vi "Update State.vi"(8 "error in (no error)":errorcluster, 11 "Car Wash Controller Actor in":refnum<class "Car Wash Controller Actor.lvclass">) -> (0 "error out":errorcluster, 3 "Car Wash Controller Actor out":refnum<class "Car Wash Controller Actor.lvclass">)   [LabVIEW 2019]
uses:
  <vilib>/ActorFramework/Actor/Actor.lvclass
  Simulated Wash Display Console Actor/Simulated Wash Display Console Actor/Simulated Wash Display Console Actor.lvclass
  Sim Entry Console Actor/Sim Entry Console Actor/Wash steps selection -Buttons.ctl
  Sim Entry Console Actor/Sim Entry Console Actor/Simulated Entry Console Actor.lvclass
  Vehicle Position Simulation/Vehicle Position Simulation/Vehicle Position Simulation.lvclass
  Car Wash Controller Actor Messages/Set State Msg/Set State Msg.lvclass
  State -Enum.ctl
  Car Wash Controller Actor.lvclass
  C:/Program Files (x86)/National Instruments/LabVIEW 2019/vi.lib/ActorFramework/Actor/Actor.lvclass
  C:/Workspace/CLA/Carwasher AF/Abstract Entry Console Actor/Abstract Entry Console Actor/Entry Console Actor.lvclass
  C:/Workspace/CLA/Carwasher AF/Abstract Washer Display Console Actor/Abstract Washer Display Console Actor/Washer Display Console Actor.lvclass
  C:/Workspace/CLA/Carwasher AF/Abstract Vehicle Position Interface/Abstract Vehicle Position Interface/Vehicle Position Interface.lvclass
  Simulated Configuration Database Actor/Simulated Configuration Database Actor/Simulated Configuration Database Actor.lvclass
  C:/Workspace/CLA/Carwasher AF/Configuration Database Actor/Configuration Database Actor/Configuration Database Actor.lvclass
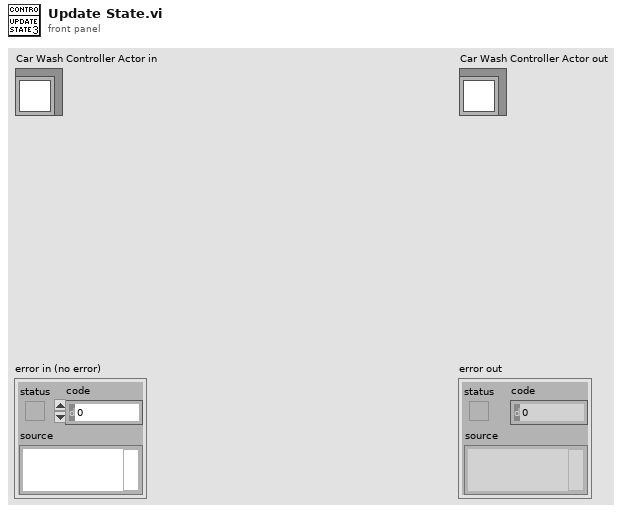
[diagram p1: front panel]
types:
  T1 = typedef "Car Wash Controller Actor.lvlib/Car Wash Controller Actor.lvclass/State -Enum.ctl" = enum16{"Initial", "Wait for Start", "Start", "Wait for Vehicle Position", "Wash Step Execution", "Wash Step/Cycle Completion", "Wash Exit", "Wash Abort/Terminate"}
  T2 = typedef "Simulated Entry Console Actor.lvlib/Simulated Entry Console Actor.lvclass/Wash steps selection -Buttons.ctl" = cluster{"Under Body Wash":bool, "Bug Remover":bool, "Pre-Soak":bool, "High Pressure Wash (default)":bool, "Low Pressure Wax":bool, "Spot Free Rinse":bool, "Tire Shine Foam":bool, "Air Dry":bool}
  T3 = enum8{"Enabled", "Disabled", "Disabled and Grayed Out"}
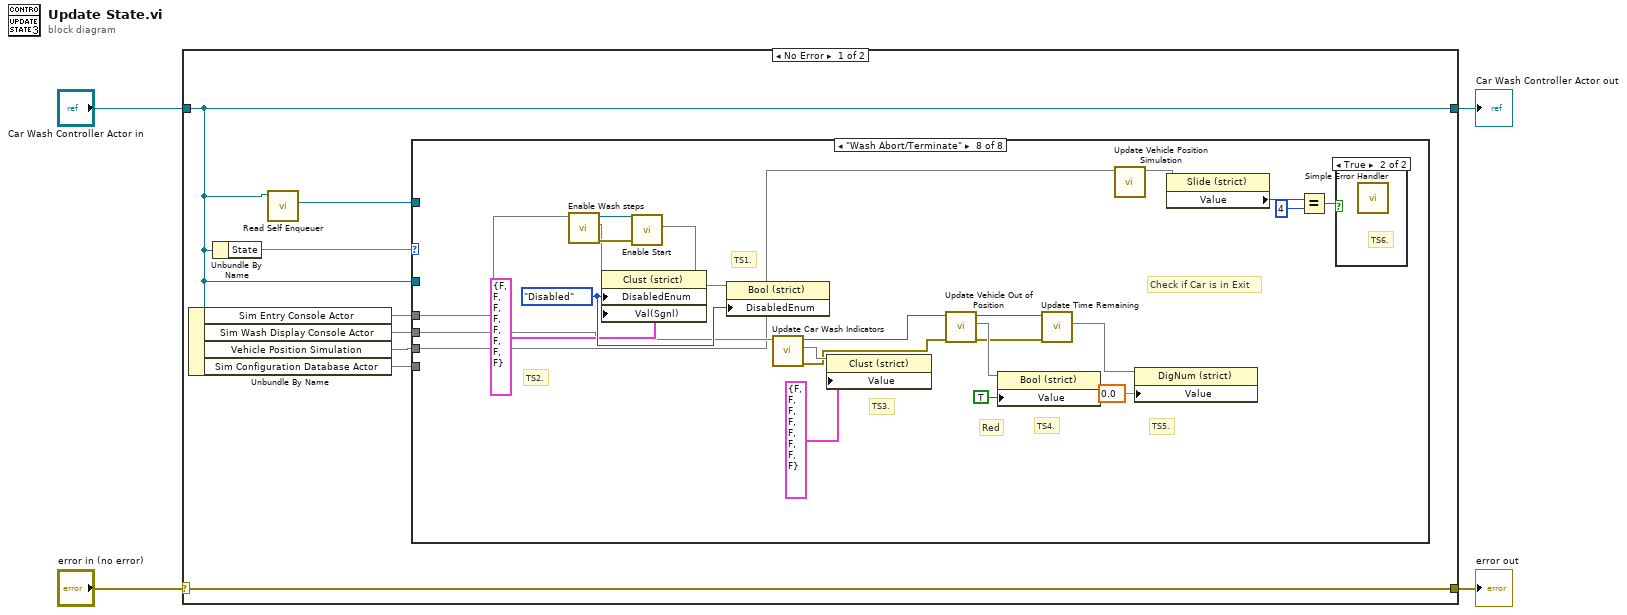
[diagram p0: block diagram]
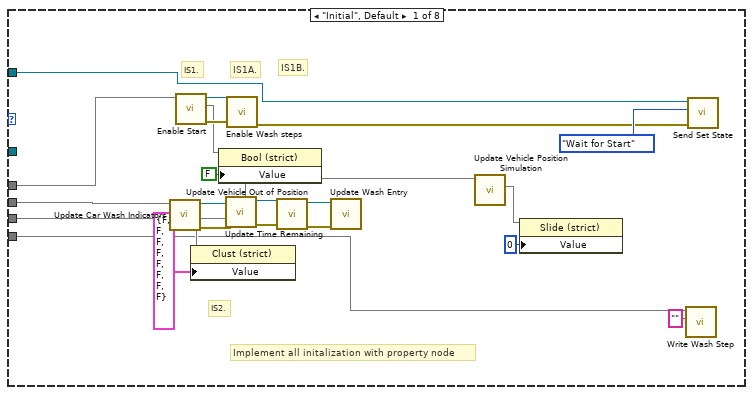
[diagram p2: hidden frame]
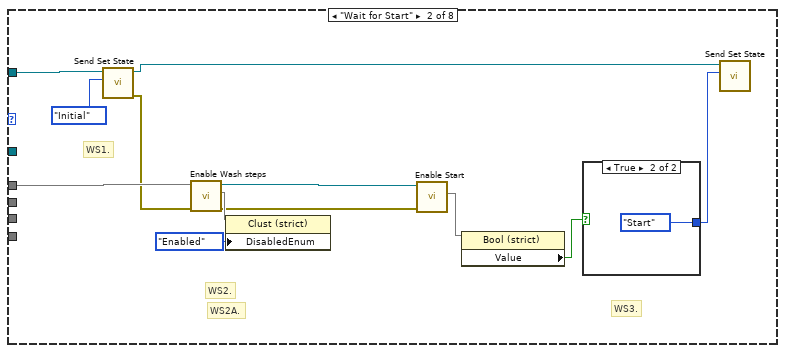
[diagram p3: hidden frame]
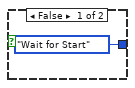
[diagram p4: hidden frame]
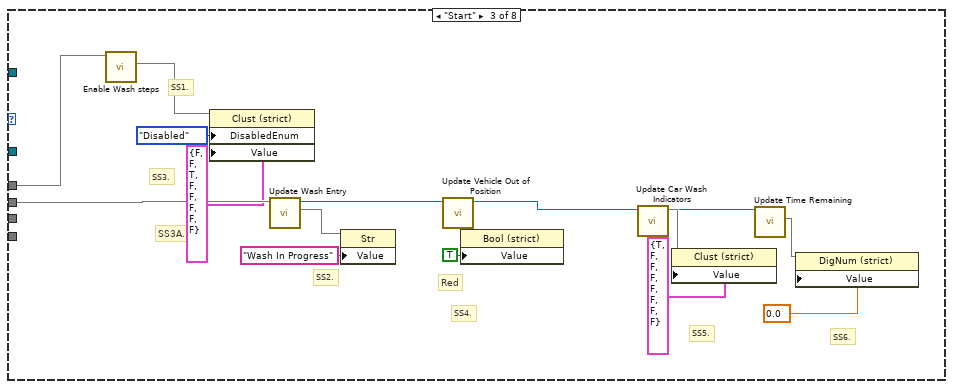
[diagram p5: hidden frame]
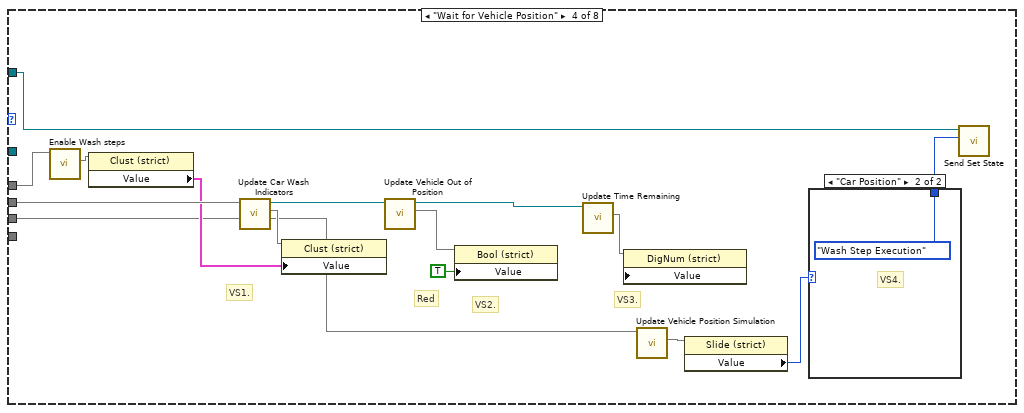
[diagram p6: hidden frame]
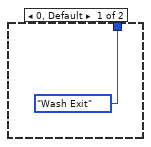
[diagram p7: hidden frame]
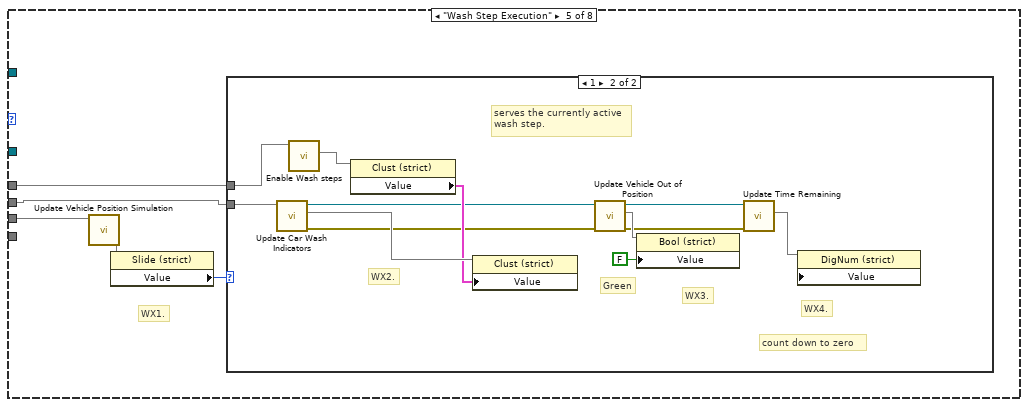
[diagram p8: hidden frame]
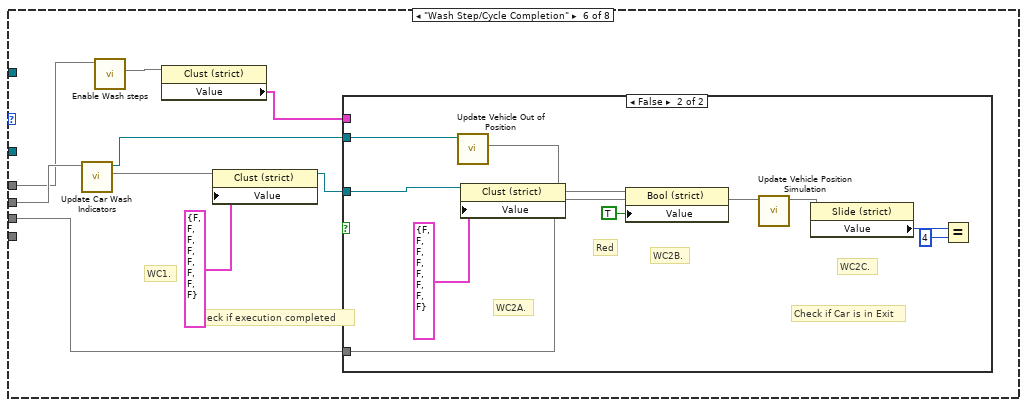
[diagram p10: hidden frame]
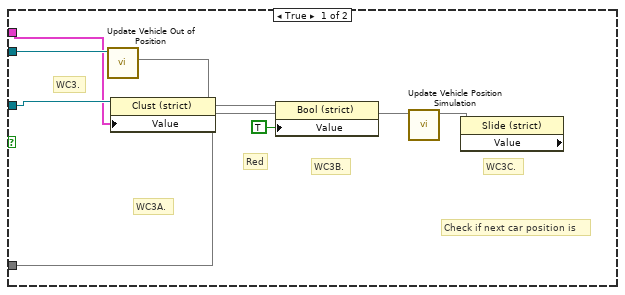
[diagram p11: hidden frame]
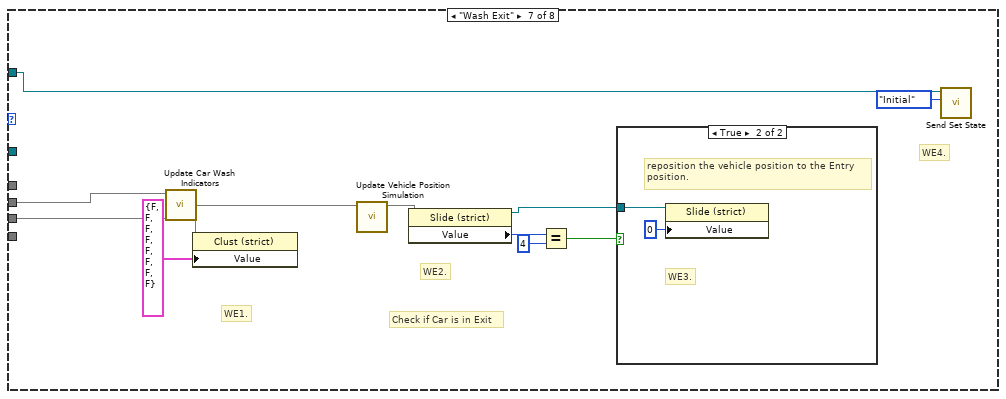
[diagram p12: hidden frame]
diagram:
  n1 = case shown="No Error" "error in (no error)" {
    selector: "error in (no error)" -> [w12 w161]
    tunnel: [w12 w161] -> w3
    tunnel: [w5 w160] -> w1
    tunnel: "Car Wash Controller Actor in" -> [w5 w160]
    frame No Error {
      n2 = Unbundle By Name(w5) -> ("Sim Entry Console Actor"=w9, "Sim Wash Display Console Actor"=w8, "Vehicle Position Simulation"=w7, "Sim Configuration Database Actor"=w6)
      n3 = Unbundle By Name(w5) -> ("State"=w11)
      n4 = call <vilib>:"Read Self Enqueuer.vi"("Actor"=w5) -> ("Self Enqueuer"=w10:refnum<class "Message Enqueuer.lvclass">)  [unwired: 10 in]
      n5 = case shown="\"Wash Abort/Terminate\"" w11 {
        tunnel: w10 -> [w15 w46 _ w66 _ _ w125 _]
        tunnel: w9 -> [w23 w44 w64 w77 w82 w101 _ w157]
        tunnel: w8 -> [w34 _ w61 w79 w83 w106 w134 w152]
        tunnel: w7 -> [w20 _ _ w69 w86 w102 w128 w138]
        tunnel: w6 -> [w17 _ _ _ _ _ _ _]
        tunnel: w5 -> [_ _ _ _ _ _ _ _]
        frame "Initial", Default {
          # "IS2."
          # "Implement all initalization with property node"
          # "IS1B."
          # "IS1A."
          # "IS1."
          n6 = call "Update Car Wash Indicators.vi"("Simulated Wash Display Console Actor in"=w34) -> ("error out"=w30:errorcluster, 2:w27, "Simulated Wash Display Console Actor out"=w33:refnum<class "Simulated Wash Display Console Actor.lvclass">)  [unwired: 8 in]
          n7 = call "Enable Start.vi"("Simulated Entry Console Actor in"=w23) -> ("error out"=w24:errorcluster, 2:w22, "Simulated Entry Console Actor out"=w25:refnum<class "Simulated Entry Console Actor.lvclass">)  [unwired: 8 in]
          n8 = property class="Clust (strict)"(reference=w27, "Value"=T2 {"Under Body Wash"=FALSE, "Bug Remover"=FALSE, "Pre-Soak"=FALSE, "High Pressure Wash (default)"=FALSE, "Low Pressure Wax"=FALSE, "Spot Free Rinse"=FALSE, "Tire Shine Foam"=FALSE, "Air Dry"=FALSE}) -> ()  [unwired: 1 in, 2 out]
          n9 = property class="Bool (strict)"(reference=w22, "Value"=FALSE) -> ()  [unwired: 1 in, 2 out]
          n10 = call "Update Time Remaining.vi"("error in (no error)"=w30, "Simulated Wash Display Console Actor in"=w33) -> ("error out"=w29:errorcluster, "Simulated Wash Display Console Actor out"=w32:refnum<class "Simulated Wash Display Console Actor.lvclass">)  [unwired: 8 in]
          n11 = call "Enable Wash steps.vi"("error in (no error)"=w24, "Simulated Entry Console Actor in"=w25) -> ("error out"=w13:errorcluster)  [unwired: 8 in, 1 out]
          n12 = call "Update Vehicle Out of Position.vi"("error in (no error)"=w29, "Simulated Wash Display Console Actor in"=w32) -> ("error out"=w28:errorcluster, "Simulated Wash Display Console Actor out"=w31:refnum<class "Simulated Wash Display Console Actor.lvclass">)  [unwired: 8 in]
          n13 = call "Update Wash Entry.vi"("error in (no error)"=w28, "Simulated Wash Display Console Actor in"=w31) -> ()  [unwired: 8 in, 2 out]
          n14 = call "Update Vehicle Position Simulation.vi"("Vehicle Position Simulation in"=w20) -> (2:w19)  [unwired: 8 in, 2 out]
          n15 = property class="Slide (strict)"(reference=w19, "Value"=u32 0) -> ()  [unwired: 1 in, 2 out]
          n16 = call-dynamic "Write Wash Step.vi"("Wash Step"="", "Simulated Configuration Database Actor in"=w17) -> ()  [unwired: 8 in, 2 out]
          n17 = call "Send Set State.vi"("error in (no error)"=w13, "States"=State_-Enum."Wait for Start", "Message Enqueuer"=w15) -> ()  [unwired: 7 in, 2 out]
        }
        frame "Wait for Start" {
          # "WS3."
          # "WS2A."
          # "WS2."
          # "WS1."
          n18 = call "Send Set State.vi"("States"=State_-Enum."Initial", "Message Enqueuer"=w46) -> ("error out"=w38:errorcluster, "Message Enqueuer out"=w36:refnum<class "Message Enqueuer.lvclass">)  [unwired: 8 in]
          n19 = call "Enable Wash steps.vi"("error in (no error)"=w38, "Simulated Entry Console Actor in"=w44) -> ("error out"=w37:errorcluster, 2:w43, "Simulated Entry Console Actor out"=w41:refnum<class "Simulated Entry Console Actor.lvclass">)  [unwired: 7 in]
          n20 = property class="Clust (strict)"(reference=w43, "DisabledEnum"=T3."Enabled" ("Disabled")) -> ()  [unwired: 1 in, 2 out]
          n21 = call "Enable Start.vi"("error in (no error)"=w37, "Simulated Entry Console Actor in"=w41) -> (2:w40)  [unwired: 7 in, 2 out]
          n22 = property class="Bool (strict)"(reference=w40) -> ("Value"=w39:bool)  [unwired: 1 in, 2 out]
          n23 = case shown="True" w39 {
            tunnel: [State_-Enum."Wait for Start" ("States") State_-Enum."Start" ("States")] -> w35
            frame False {
            }
            frame True {
            }
          }
          n24 = call "Send Set State.vi"("States"=w35, "Message Enqueuer"=w36) -> ()  [unwired: 8 in, 2 out]
        }
        frame "Start" {
          # "SS6."
          # "SS5."
          # "SS4."
          # "Red"
          # "SS3A."
          # "SS3."
          # "SS2."
          # "SS1."
          n25 = call "Enable Wash steps.vi"("Simulated Entry Console Actor in"=w64) -> (2:w63)  [unwired: 8 in, 2 out]
          n26 = property class="Clust (strict)"(reference=w63, "DisabledEnum"=T3."Disabled" ("Disabled"), "Value"=T2 {"Under Body Wash"=FALSE, "Bug Remover"=FALSE, "Pre-Soak"=TRUE, "High Pressure Wash (default)"=FALSE, "Low Pressure Wax"=FALSE, "Spot Free Rinse"=FALSE, "Tire Shine Foam"=FALSE, "Air Dry"=FALSE}) -> ()  [unwired: 1 in, 2 out]
          n27 = call "Update Wash Entry.vi"("Simulated Wash Display Console Actor in"=w61) -> (2:w60, "Simulated Wash Display Console Actor out"=w57:refnum<class "Simulated Wash Display Console Actor.lvclass">)  [unwired: 8 in, 1 out]
          n28 = property class="Str"(reference=w60, "Value"="Wash In Progress") -> ()  [unwired: 1 in, 2 out]
          n29 = call "Update Vehicle Out of Position.vi"("Simulated Wash Display Console Actor in"=w57) -> (2:w56, "Simulated Wash Display Console Actor out"=w54:refnum<class "Simulated Wash Display Console Actor.lvclass">)  [unwired: 8 in, 1 out]
          n30 = property class="Bool (strict)"(reference=w56, "Value"=TRUE) -> ()  [unwired: 1 in, 2 out]
          n31 = call "Update Car Wash Indicators.vi"("Simulated Wash Display Console Actor in"=w54) -> (2:w53, "Simulated Wash Display Console Actor out"=w51:refnum<class "Simulated Wash Display Console Actor.lvclass">)  [unwired: 8 in, 1 out]
          n32 = property class="Clust (strict)"(reference=w53, "Value"=T2 {"Under Body Wash"=TRUE, "Bug Remover"=FALSE, "Pre-Soak"=FALSE, "High Pressure Wash (default)"=FALSE, "Low Pressure Wax"=FALSE, "Spot Free Rinse"=FALSE, "Tire Shine Foam"=FALSE, "Air Dry"=FALSE}) -> ()  [unwired: 1 in, 2 out]
          n33 = call "Update Time Remaining.vi"("Simulated Wash Display Console Actor in"=w51) -> (2:w50)  [unwired: 8 in, 2 out]
          n34 = property class="DigNum (strict)"(reference=w50, "Value"=0.0) -> ()  [unwired: 1 in, 2 out]
        }
        frame "Wait for Vehicle Position" {
          # "VS3."
          # "VS2."
          # "Red"
          # "VS1."
          n35 = call "Enable Wash steps.vi"("Simulated Entry Console Actor in"=w77) -> (2:w76)  [unwired: 8 in, 2 out]
          n36 = property class="Clust (strict)"(reference=w76) -> ("Value"=w75:T2)  [unwired: 1 in, 2 out]
          n37 = call "Update Car Wash Indicators.vi"("Simulated Wash Display Console Actor in"=w79) -> (2:w78, "Simulated Wash Display Console Actor out"=w74:refnum<class "Simulated Wash Display Console Actor.lvclass">)  [unwired: 8 in, 1 out]
          n38 = property class="Clust (strict)"(reference=w78, "Value"=w75) -> ()  [unwired: 1 in, 2 out]
          n39 = call "Update Vehicle Out of Position.vi"("Simulated Wash Display Console Actor in"=w74) -> (2:w73, "Simulated Wash Display Console Actor out"=w71:refnum<class "Simulated Wash Display Console Actor.lvclass">)  [unwired: 8 in, 1 out]
          n40 = property class="Bool (strict)"(reference=w73, "Value"=TRUE) -> ()  [unwired: 1 in, 2 out]
          n41 = call "Update Time Remaining.vi"("Simulated Wash Display Console Actor in"=w71) -> (2:w70)  [unwired: 8 in, 2 out]
          n42 = property class="DigNum (strict)" props=["Value"](reference=w70) -> ()  [unwired: 2 in, 2 out]
          n43 = call "Update Vehicle Position Simulation.vi"("Vehicle Position Simulation in"=w69) -> (2:w68)  [unwired: 8 in, 2 out]
          n44 = property class="Slide (strict)"(reference=w68) -> ("Value"=w67:u32)  [unwired: 1 in, 2 out]
          n45 = case shown="\"Car Position\"" w67 {
            tunnel: [State_-Enum."Wash Exit" ("States") State_-Enum."Wash Step Execution" ("States")] -> w65
            frame 0, Default {
            }
            frame 0 {
              # "VS4."
            }
          }
          n46 = call "Send Set State.vi"("States"=w65, "Message Enqueuer"=w66) -> ()  [unwired: 8 in, 2 out]
        }
        frame "Wash Step Execution" {
          # "WX1."
          n47 = call "Update Vehicle Position Simulation.vi"("Vehicle Position Simulation in"=w86) -> (2:w85)  [unwired: 8 in, 2 out]
          n48 = property class="Slide (strict)"(reference=w85) -> ("Value"=w84:u32)  [unwired: 1 in, 2 out]
          n49 = case shown="1" w84 {
            tunnel: w83 -> [_ w98]
            tunnel: w82 -> [_ w96]
            frame 0, Default {
            }
            frame 1 {
              # "count down to zero"
              # "WX4."
              # "Green"
              # "WX3."
              # "serves the currently active\nwash step."
              # "WX2."
              n50 = call "Update Car Wash Indicators.vi"("Simulated Wash Display Console Actor in"=w98) -> ("error out"=w89:errorcluster, 2:w97, "Simulated Wash Display Console Actor out"=w93:refnum<class "Simulated Wash Display Console Actor.lvclass">)  [unwired: 8 in]
              n51 = call "Enable Wash steps.vi"("Simulated Entry Console Actor in"=w96) -> (2:w95)  [unwired: 8 in, 2 out]
              n52 = property class="Clust (strict)"(reference=w95) -> ("Value"=w94:T2)  [unwired: 1 in, 2 out]
              n53 = property class="Clust (strict)"(reference=w97, "Value"=w94) -> ()  [unwired: 1 in, 2 out]
              n54 = call "Update Vehicle Out of Position.vi"("error in (no error)"=w89, "Simulated Wash Display Console Actor in"=w93) -> ("error out"=w88:errorcluster, 2:w92, "Simulated Wash Display Console Actor out"=w90:refnum<class "Simulated Wash Display Console Actor.lvclass">)  [unwired: 7 in]
              n55 = property class="Bool (strict)"(reference=w92, "Value"=FALSE) -> ()  [unwired: 1 in, 2 out]
              n56 = call "Update Time Remaining.vi"("error in (no error)"=w88, "Simulated Wash Display Console Actor in"=w90) -> (2:w87)  [unwired: 7 in, 2 out]
              n57 = property class="DigNum (strict)" props=["Value"](reference=w87) -> ()  [unwired: 2 in, 2 out]
            }
          }
        }
        frame "Wash Step/Cycle Completion" {
          # "Check if execution completed"
          # "WC1."
          n58 = call "Update Car Wash Indicators.vi"("Simulated Wash Display Console Actor in"=w106) -> (2:w107, "Simulated Wash Display Console Actor out"=w103:refnum<class "Simulated Wash Display Console Actor.lvclass">)  [unwired: 8 in, 1 out]
          n59 = call "Enable Wash steps.vi"("Simulated Entry Console Actor in"=w101) -> (2:w100)  [unwired: 8 in, 2 out]
          n60 = property class="Clust (strict)"(reference=w100) -> ("Value"=w99:T2)  [unwired: 1 in, 2 out]
          n61 = property class="Clust (strict)"(reference=w107, "Value"=T2 {"Under Body Wash"=FALSE, "Bug Remover"=FALSE, "Pre-Soak"=FALSE, "High Pressure Wash (default)"=FALSE, "Low Pressure Wax"=FALSE, "Spot Free Rinse"=FALSE, "Tire Shine Foam"=FALSE, "Air Dry"=FALSE}) -> (reference out=w104:refnum<vi>)  [unwired: 1 in, 1 out]
          n62 = case shown="\"Last Step\"" {
            selector: _ -> [_ _]
            tunnel: w104 -> [w110 w123]
            tunnel: w103 -> [w111 w121]
            tunnel: w102 -> [w109 w118]
            tunnel: w99 -> [w108 _]
            frame True {
              # "WC3A."
              # "WC3C."
              # "WC3B."
              # "Check if next car position is"
              # "Red"
              # "WC3."
              n63 = call "Update Vehicle Out of Position.vi"("Simulated Wash Display Console Actor in"=w111) -> (2:w114)  [unwired: 8 in, 2 out]
              n64 = property class="Clust (strict)"(reference=w110, "Value"=w108) -> ()  [unwired: 1 in, 2 out]
              n65 = property class="Bool (strict)"(reference=w114, "Value"=TRUE) -> ()  [unwired: 1 in, 2 out]
              n66 = call "Update Vehicle Position Simulation.vi"("Vehicle Position Simulation in"=w109) -> (2:w112)  [unwired: 8 in, 2 out]
              n67 = property class="Slide (strict)" props=["Value"](reference=w112) -> ()  [unwired: 1 in, 3 out]
            }
            frame False {
              # "Check if Car is in Exit"
              # "WC2C."
              # "WC2B."
              # "Red"
              # "WC2A."
              n68 = call "Update Vehicle Out of Position.vi"("Simulated Wash Display Console Actor in"=w121) -> (2:w120)  [unwired: 8 in, 2 out]
              n69 = property class="Clust (strict)"(reference=w123, "Value"=T2 {"Under Body Wash"=FALSE, "Bug Remover"=FALSE, "Pre-Soak"=FALSE, "High Pressure Wash (default)"=FALSE, "Low Pressure Wax"=FALSE, "Spot Free Rinse"=FALSE, "Tire Shine Foam"=FALSE, "Air Dry"=FALSE}) -> ()  [unwired: 1 in, 2 out]
              n70 = property class="Bool (strict)"(reference=w120, "Value"=TRUE) -> ()  [unwired: 1 in, 2 out]
              n71 = call "Update Vehicle Position Simulation.vi"("Vehicle Position Simulation in"=w118) -> (2:w117)  [unwired: 8 in, 2 out]
              n72 = property class="Slide (strict)"(reference=w117) -> ("Value"=w116:u32)  [unwired: 1 in, 2 out]
              n73 = Equal?(x=w116, y=u32 4) -> ()  [unwired: 1 out]
            }
          }
        }
        frame "Wash Exit" {
          # "WE4."
          # "WE2."
          # "Check if Car is in Exit"
          # "WE1."
          n74 = call "Update Car Wash Indicators.vi"("Simulated Wash Display Console Actor in"=w134) -> (2:w133)  [unwired: 8 in, 2 out]
          n75 = property class="Clust (strict)"(reference=w133, "Value"=T2 {"Under Body Wash"=FALSE, "Bug Remover"=FALSE, "Pre-Soak"=FALSE, "High Pressure Wash (default)"=FALSE, "Low Pressure Wax"=FALSE, "Spot Free Rinse"=FALSE, "Tire Shine Foam"=FALSE, "Air Dry"=FALSE}) -> ()  [unwired: 1 in, 2 out]
          n76 = call "Update Vehicle Position Simulation.vi"("Vehicle Position Simulation in"=w128) -> (2:w131)  [unwired: 8 in, 2 out]
          n77 = property class="Slide (strict)"(reference=w131) -> (reference out=w126:refnum<vi>, "Value"=w130:u32)  [unwired: 1 in, 1 out]
          n78 = Equal?(x=w130, y=u32 4) -> (x = y?=w127:bool)
          n79 = case shown="True" w127 {
            tunnel: w126 -> [_ w136]
            frame False {
            }
            frame True {
              # "reposition the vehicle position to the Entry\nposition."
              # "WE3."
              n80 = property class="Slide (strict)"(reference=w136, "Value"=u32 0) -> ()  [unwired: 1 in, 2 out]
            }
          }
          n81 = call "Send Set State.vi"("States"=State_-Enum."Initial", "Message Enqueuer"=w125) -> ()  [unwired: 8 in, 2 out]
        }
        frame "Wash Abort/Terminate" {
          w154 = T3."Disabled" ("Disabled")
          # "Check if Car is in Exit"
          # "TS5."
          # "TS4."
          # "Red"
          # "TS3."
          # "TS2."
          # "TS1."
          n82 = call "Enable Wash steps.vi"("Simulated Entry Console Actor in"=w157) -> ("error out"=w158:errorcluster, 2:w156, "Simulated Entry Console Actor out"=w159:refnum<class "Simulated Entry Console Actor.lvclass">)  [unwired: 8 in]
          n83 = property class="Clust (strict)"(reference=w156, "DisabledEnum"=w154, "Val(Sgnl)"=T2 {"Under Body Wash"=FALSE, "Bug Remover"=FALSE, "Pre-Soak"=FALSE, "High Pressure Wash (default)"=FALSE, "Low Pressure Wax"=FALSE, "Spot Free Rinse"=FALSE, "Tire Shine Foam"=FALSE, "Air Dry"=FALSE} ("Value")) -> ()  [unwired: 1 in, 2 out]
          n84 = call "Enable Start.vi"("error in (no error)"=w158, "Simulated Entry Console Actor in"=w159) -> (2:w155)  [unwired: 7 in, 2 out]
          n85 = property class="Bool (strict)"(reference=w155, "DisabledEnum"=w154) -> ()  [unwired: 1 in, 2 out]
          n86 = call "Update Car Wash Indicators.vi"("Simulated Wash Display Console Actor in"=w152) -> ("error out"=w148:errorcluster, 2:w151, "Simulated Wash Display Console Actor out"=w149:refnum<class "Simulated Wash Display Console Actor.lvclass">)  [unwired: 8 in]
          n87 = property class="Clust (strict)"(reference=w151, "Value"=T2 {"Under Body Wash"=FALSE, "Bug Remover"=FALSE, "Pre-Soak"=FALSE, "High Pressure Wash (default)"=FALSE, "Low Pressure Wax"=FALSE, "Spot Free Rinse"=FALSE, "Tire Shine Foam"=FALSE, "Air Dry"=FALSE}) -> ()  [unwired: 1 in, 2 out]
          n88 = call "Update Vehicle Out of Position.vi"("error in (no error)"=w148, "Simulated Wash Display Console Actor in"=w149) -> ("error out"=w144:errorcluster, 2:w147, "Simulated Wash Display Console Actor out"=w145:refnum<class "Simulated Wash Display Console Actor.lvclass">)  [unwired: 7 in]
          n89 = property class="Bool (strict)"(reference=w147, "Value"=TRUE) -> ()  [unwired: 1 in, 2 out]
          n90 = call "Update Time Remaining.vi"("error in (no error)"=w144, "Simulated Wash Display Console Actor in"=w145) -> (2:w143)  [unwired: 7 in, 2 out]
          n91 = call "Update Vehicle Position Simulation.vi"("Vehicle Position Simulation in"=w138) -> (2:w141)  [unwired: 8 in, 2 out]
          n92 = property class="DigNum (strict)"(reference=w143, "Value"=0.0) -> ()  [unwired: 1 in, 2 out]
          n93 = property class="Slide (strict)"(reference=w141) -> ("Value"=w140:u32)  [unwired: 1 in, 2 out]
          n94 = Equal?(x=w140, y=u32 4) -> (x = y?=w137:bool)
          n95 = case shown="True" w137 {
            frame False {
            }
            frame True {
              # "TS6."
              n96 = call <vilib>:"Simple Error Handler.vi"() -> ()  [unwired: 5 in, 5 out]
            }
          }
        }
      }
    }
    frame Error {
    }
  }
  "error out" <- w3
  "Car Wash Controller Actor out" <- w1
